vi "MIMIC Port.vi"(0 "VISA resource name":refnum<visa-resource-name>, 1 "Port Setting":T1={"timeout"=10000, "baud rate"=9600, "data bits"=8, "parity (0:none)"=enum."None", "stop bits (10: 1 bit)"=10} {"stop bits (10: 1 bit)" items=["1.0"=10, "1.5"=15, "2.0"=20]; "data bits" min=5 max=8 step=1}, 2 "write buffer":string, 5 "error in (no error)":errorcluster, 6 "Function":T2(ring)) -> (14 "output VISA resource name":refnum<visa-resource-name>, 16 "Read Buffer":string, 18 "return count":u32, 19 "error out":errorcluster)   [LabVIEW 2014]
uses:
  <vilib>/Instr/_visa.llb/VISA Flush IO Buffer Mask.ctl
  <vilib>/Instr/_visa.llb/VISA Configure Serial Port (Instr).vi
panel:
  # "MIMIC PORT"
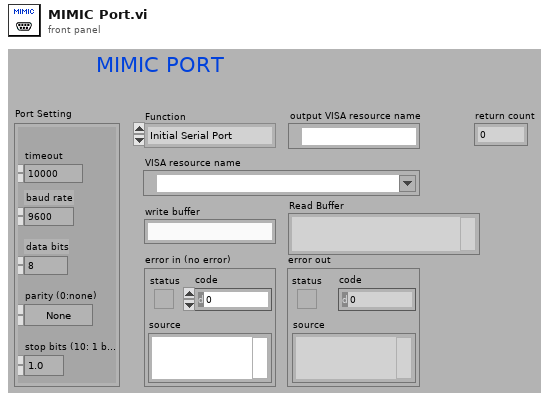
[diagram p1: front panel]
types:
  T1 = cluster{"timeout":u32, "baud rate":u32, "data bits":u16, "parity (0:none)":enum16{"None", "Odd", "Even", "Mark", "Space"}, "stop bits (10: 1 bit)":u16}
  T2 = enum16{"Initial Serial Port", "Write", "Read", "Close", "ClearBuff"}
  T3 = typedef "VISA Flush IO Buffer Mask.ctl" = u16
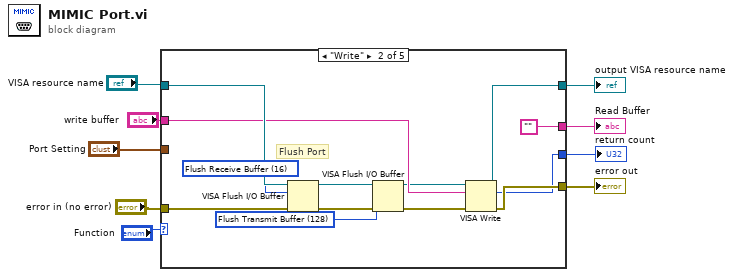
[diagram p0: block diagram]
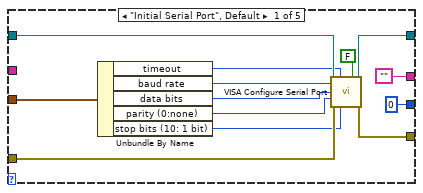
[diagram p2: hidden frame]
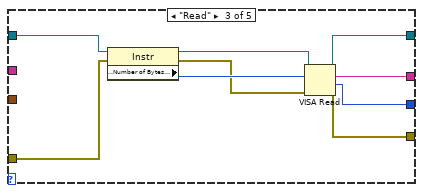
[diagram p3: hidden frame]
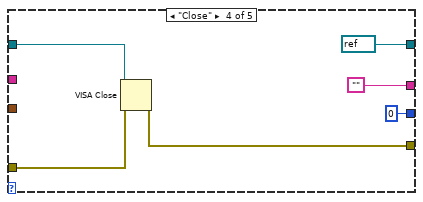
[diagram p4: hidden frame]
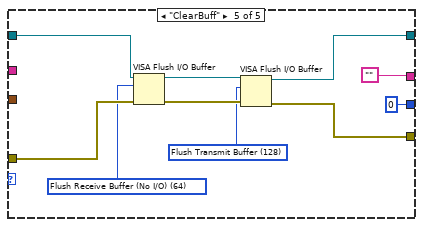
[diagram p5: hidden frame]
diagram:
  n1 = case shown="\"Write\"" "Function" {
    tunnel: "VISA resource name" -> [w19 w31 w41 w49 w55]
    tunnel: "Port Setting" -> [w22 _ _ _ _]
    tunnel: "error in (no error)" -> [w21 w30 w39 w50 w56]
    tunnel: [w20 w35 w44 w48 w57] -> w5
    tunnel: "write buffer" -> [_ w29 _ _ _]
    tunnel: ["" "" w43 "" ""] -> w6
    tunnel: [w17 w33 w42 refnum<visa-resource-name> refnum ("VISA resource name") w54] -> w3
    tunnel: [u32 0 ("return count") w32 w36 u32 0 ("return count") u32 0 ("return count")] -> w2
    frame "Initial Serial Port", Default {
      n2 = Unbundle By Name(w22) -> ("timeout"=w14:u32, "baud rate"=w13:u32, "data bits"=w12:u16, "parity (0:none)"=w11:enum16{"None", "Odd", "Even", "Mark", "Space"}, "stop bits (10: 1 bit)"=w10:u16)
      n3 = call-poly "VISA Configure Serial Port"("VISA resource name"=w19, "timeout (10sec)"=w14, "Enable Termination\nChar (T)"=FALSE ("Enable Termination\nChar (T)"), "baud rate (9600)"=w13, "data bits (8)"=w12, "parity (0:none)"=w11, "error in (no error)"=w21, "stop bits (10: 1 bit)"=w10) -> ("VISA resource name out"=w17:refnum<visa-resource-name>, "error out"=w20:errorcluster)  [unwired: 6 in]
    }
    frame "Write" {
      w25 = T3 128 items=["Flush Receive Buffer"=16, "Write Transmit Buffer to Device"=32, "Flush Receive Buffer (No I/O)"=64, "Flush Transmit Buffer"=128] ("Mask")
      w28 = T3 16 items=["Flush Receive Buffer"=16, "Write Transmit Buffer to Device"=32, "Flush Receive Buffer (No I/O)"=64, "Flush Transmit Buffer"=128] ("Mask")
      # "Flush Port"
      n4 = VISA Flush I/O Buffer(VISA resource name=w31, mask (16)=w28, error in (no error)=w30) -> (VISA resource name out=w27:refnum<visa-resource-name>, error out=w24:errorcluster)
      n5 = VISA Flush I/O Buffer(VISA resource name=w27, mask (16)=w25, error in (no error)=w24) -> (VISA resource name out=w26:refnum<visa-resource-name>, error out=w23:errorcluster)
      n6 = VISA Write(VISA resource name=w26, write buffer=w29, error in (no error)=w23) -> (VISA resource name out=w33:refnum<visa-resource-name>, return count=w32:u32, error out=w35:errorcluster)
    }
    frame "Read" {
      n7 = property class="Instr"(reference=w41, error in=w39) -> (reference out=w40:refnum<visa-resource-name>, error out=w37:errorcluster, "Serial Settings:Number of Bytes at Serial Port"=w38:u32)
      n8 = VISA Read(VISA resource name=w40, byte count=w38, error in (no error)=w37) -> (VISA resource name out=w42:refnum<visa-resource-name>, read buffer=w43:string, return count=w36:u32, error out=w44:errorcluster)
    }
    frame "Close" {
      n9 = VISA Close(VISA resource name=w49, error in (no error)=w50) -> (error out=w48:errorcluster)
    }
    frame "ClearBuff" {
      w52 = T3 128 items=["Flush Receive Buffer"=16, "Write Transmit Buffer to Device"=32, "Flush Receive Buffer (No I/O)"=64, "Flush Transmit Buffer"=128] ("Mask")
      w53 = T3 64 items=["Flush Receive Buffer"=16, "Write Transmit Buffer to Device"=32, "Flush Receive Buffer (No I/O)"=64, "Flush Transmit Buffer"=128] ("Mask")
      n10 = VISA Flush I/O Buffer(VISA resource name=w55, mask (16)=w53, error in (no error)=w56) -> (VISA resource name out=w59:refnum<visa-resource-name>, error out=w58:errorcluster)
      n11 = VISA Flush I/O Buffer(VISA resource name=w59, mask (16)=w52, error in (no error)=w58) -> (VISA resource name out=w54:refnum<visa-resource-name>, error out=w57:errorcluster)
    }
  }
  "error out" <- w5
  "Read Buffer" <- w6
  "output VISA resource name" <- w3
  "return count" <- w2
